vi "LVDimInterface.dim_semaphore.vi"(3 "Action":T2(ring)) -> (17 "semaphore":T1)   [LabVIEW 2014, in "LVDimInterface.lvlib"]
doc: "This VI represents a functional global variable providing the semaphore that is used for the LVDimInterface\n\nHistory: 03-MAR-2006, Dietrich Beck\n\nCopyright (C)\nGesellschaft für Schwerionenforschung, GSI\nPlanckstr. 1\n64291 Darmstadt\nGermany\n\nContact: D.Beck@gsi.de \n\nThis program is free software; you can redistribute it and/or modify it under the terms of the \nGNU General Public License as published by the Free Software Foundation; either version 2 of the license, or (at your option) any later version.\n\nThis program is distributed in the hope that it will be useful, but WITHOUT ANY WARRANTY; without even the implied warranty of MERCHANTABILITY or FITNESS FOR A PARTICULAR PURPOSE. See the GNU General License for more details (http://www.gnu.org).\n\nGesellschaft für Schwerionenforschung, GSI\nPlanckstr. 1, 64291 Darmstadt, Germany\nFor all questions and ideas contact D. Beck.\nLast update: 16-DEC-2005"
uses:
  LVDimInterface.lvlib
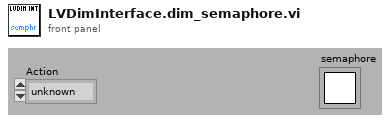
[diagram p1: front panel]
types:
  T1 = typedef "Semaphore RefNum" = refnum<k1>
  T2 = enum16{"unknown", "createSemaphore", "destroySemaphore", "getSemaphore"}
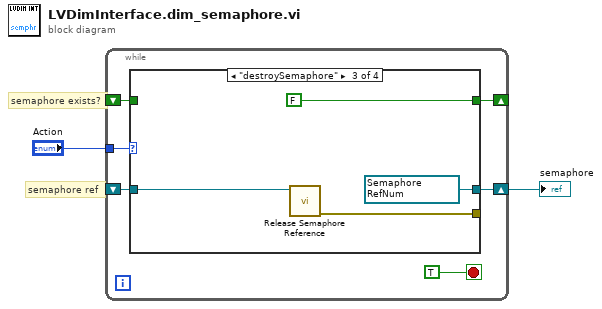
[diagram p0: block diagram]
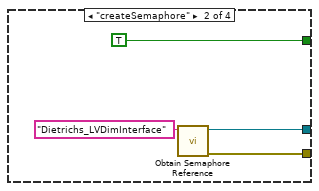
[diagram p3: hidden frame]
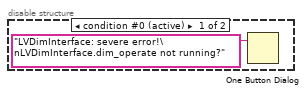
[diagram p6: hidden frame]
diagram:
  # "semaphore ref"
  # "semaphore exists?"
  n1 = while {
    tunnel: "Action" -> [w7]
    shift-right: [w6] -> w1
    shift-left: _ -> [w5]
    shift-right: [w4] -> _
    shift-left: _ -> [w3]
    stop <- TRUE stop-if-true
    n2 = case shown="\"destroySemaphore\"" w7 {
      tunnel: [w10 w13 w17 w20] -> w6
      tunnel: w5 -> [w10 _ w18 w20]
      tunnel: [w9 TRUE FALSE w19] -> w4
      tunnel: w3 -> [w9 _ _ w19]
      tunnel: [_ w11 w15 _] -> _
      frame "unknown", Default {
      }
      frame "createSemaphore" {
        n3 = call <vilib>:"Obtain Semaphore Reference.vi"("name (unnamed)"="Dietrichs_LVDimInterface") -> ("error out"=w11:errorcluster, "semaphore"=w13:T1)  [unwired: 4 in, 1 out]
      }
      frame "destroySemaphore" {
        w17 = T1 refnum items=["semaphore"] ("semaphore")
        n4 = call <vilib>:"Release Semaphore Reference.vi"("semaphore"=w18) -> ("error out"=w15:errorcluster)  [unwired: 9 in, 1 out]
      }
      frame "getSemaphore" {
        n5 = case shown="True" w19 {
          frame False {
            n6 = disable-structure shown="TARGET_TYPE==RT" {
              frame condition #0 (active) {
                n7 = One Button Dialog(message="LVDimInterface: severe error!\nLVDimInterface.dim_operate not running?") -> ()  [unwired: 1 in, 1 out]
              }
              frame condition #1 {
              }
            }
          }
          frame True {
          }
        }
      }
    }
  }
  "semaphore" <- w1
